vi "Configure Assert Engine.vi"(8 "error in (no error)":errorcluster, 10 "Startup Notifier":refnum<notifier>) -> (0 "error out":errorcluster, 3 "AssertEngine out":refnum<class "AssertEngine.lvclass">)   [LabVIEW 2016, in "AssertEngine.lvlib" / "AssertEngine.lvclass"]
uses:
  AssertEngine.lvclass
  AssertEngine.lvclass/AssertEngine.ctl
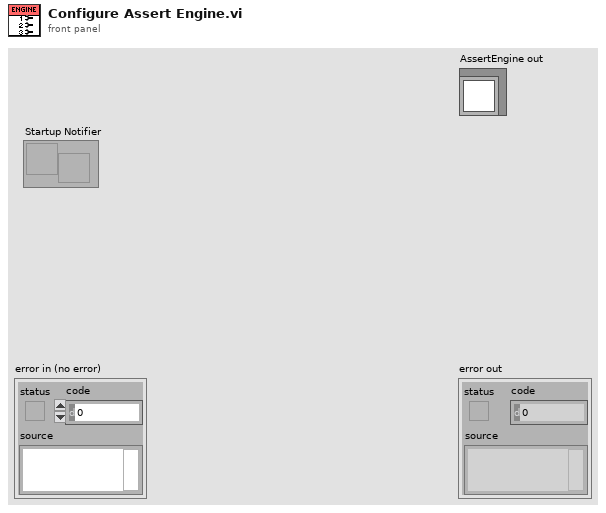
[diagram p1: front panel]
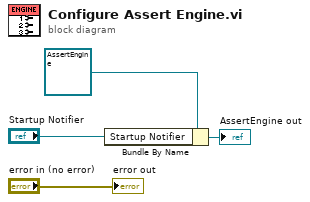
[diagram p0: block diagram]
diagram:
  n1 = Bundle By Name(cluster=refnum<class "AssertEngine.lvclass"> refnum ("AssertEngine in"), "Startup Notifier"="Startup Notifier") -> (→"AssertEngine out":refnum<class "AssertEngine.lvclass">)
  "error out" <- "error in (no error)"
